vi "MGI Restore Front Panel Data.vi"(6 "Section Name (\"Data Values\")":string="Data Values", 7 "VI (Caller)":refnum<vi>, 8 "error in (no error)":errorcluster, 11 "Path":path) -> (0 "Error Out":errorcluster)   [LabVIEW 2020]
doc: "Restores the control and indicator data from the specified MGI Read/Write Anything file.\nControl and Indicator names must be unique.\n\nAuthored by Shawn Walpole\nsupport@mooregoodideas.com\nwww.mooregoodideas.com\n\nCopyright (c) 2010, Moore Good Ideas, Inc.\n\nAll rights reserved.\n\nRedistribution and use in source and binary forms, with or without modification, are permitted provided that the following conditions are met:\n\n * Redistributions of source code must retain the above copyright notice, this list of conditions and the following disclaimer.\n * Redistributions in binary form must reproduce the above copyright notice, this list of conditions and the following disclaimer in the documentation and/or other materials provided with the distribution.\n * Neither the name of Moore Good Ideas, Inc. nor the names of its contributors may be used to endorse or promote products derived from this software without specific prior written permission.\n\nTHIS SOFTWARE IS PROVIDED BY THE COPYRIGHT HOLDERS AND CONTRIBUTORS \"AS IS\" AND ANY EXPRESS OR IMPLIED WARRANTIES, INCLUDING, BUT NOT LIMITED TO, THE IMPLIED WARRANTIES OF MERCHANTABILITY AND FITNESS FOR A PARTICULAR PURPOSE ARE DISCLAIMED. IN NO EVENT SHALL THE COPYRIGHT OWNER OR CONTRIBUTORS BE LIABLE FOR ANY DIRECT, INDIRECT, INCIDENTAL, SPECIAL, EXEMPLARY, OR CONSEQUENTIAL DAMAGES (INCLUDING, BUT NOT LIMITED TO, PROCUREMENT OF SUBSTITUTE GOODS OR SERVICES; LOSS OF USE, DATA, OR PROFITS; OR BUSINESS INTERRUPTION) HOWEVER CAUSED AND ON ANY THEORY OF LIABILITY, WHETHER IN CONTRACT, STRICT LIABILITY, OR TORT (INCLUDING NEGLIGENCE OR OTHERWISE) ARISING IN ANY WAY OUT OF THE USE OF THIS SOFTWARE, EVEN IF ADVISED OF THE POSSIBILITY OF SUCH DAMAGE."
uses:
  <userlib>/_MGI/Application Control/MGI VI Reference/MGI Caller's VI Reference.vi
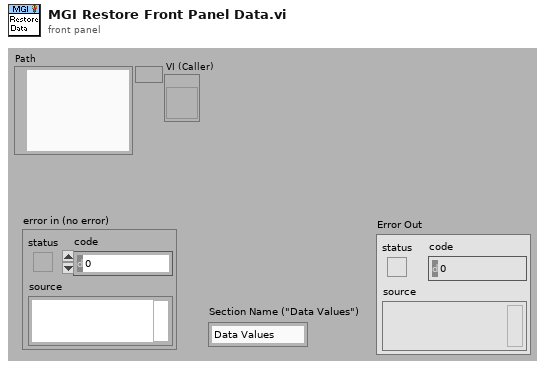
[diagram p1: front panel]
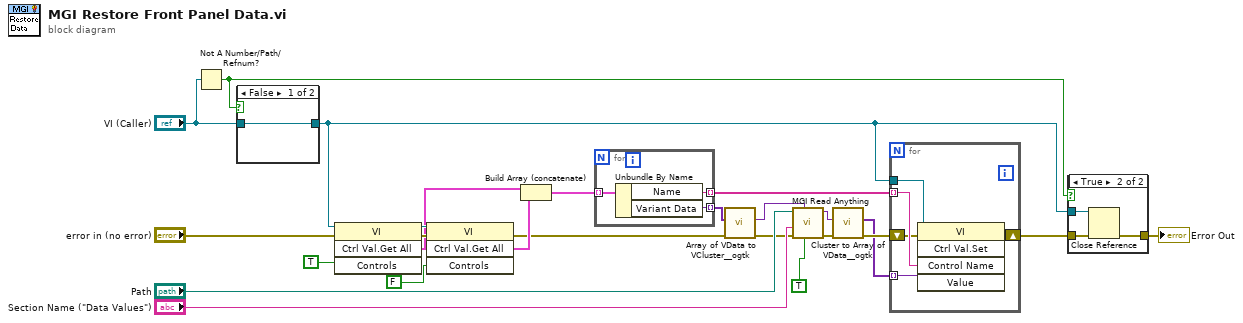
[diagram p0: block diagram]
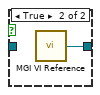
[diagram p3: hidden frame]
diagram:
  n1 = Not A Number/Path/Refnum?(number/path/refnum="VI (Caller)") -> (NaN/Path/Refnum?=w22:bool)
  n2 = case shown="False" w22 {
    tunnel: [w26 w27] -> w1
    tunnel: "VI (Caller)" -> [w26 _]
    frame False {
    }
    frame True {
      n3 = call-poly <userlib>:"MGI VI Reference.vi"() -> ("Caller's VI Reference"=w27:refnum<vi>)  [unwired: 1 in]
    }
  }
  n4 = invoke class="VI" method="Ctrl Val.Get All"(reference=w1, error in="error in (no error)", "Controls"=TRUE) -> (reference out=w18:refnum<vi>, error out=w17:errorcluster, "Get All Control Values Variant"=w16:cluster{"Name":string, "Variant Data":variant}[])  [unwired: 1 in, 1 out]
  n5 = invoke class="VI" method="Ctrl Val.Get All"(reference=w18, error in=w17, "Controls"=FALSE) -> (error out=w12:errorcluster, "Get All Control Values Variant"=w15:cluster{"Name":string, "Variant Data":variant}[])  [unwired: 1 in, 2 out]
  n6 = Build Array (concatenate)(w16, w15) -> (w11:cluster{"Name":string, "Variant Data":variant}[])
  n7 = for {
    tunnel: w11 -> [w29] mode=indexing
    tunnel: [w30] -> w3 mode=indexing
    tunnel: [w28] -> w9 mode=indexing
    n8 = Unbundle By Name(w29) -> ("Name"=w28:string, "Variant Data"=w30:variant)
  }
  n9 = call <userlib>:"Array of VData to VCluster__ogtk.vi"("error in (no error)"=w12, "Array"=w3) -> ("error out"=w4:errorcluster, "VCluster"=w5:variant)  [unwired: 8 in]
  n10 = call <userlib>:"MGI Read Anything.vi"("Use Supplied (F: Use Default)"=TRUE, "Type of Anything"=w5, "Error In"=w4, "Section Name (Name of \"Type of Anything\")"="Section Name (\"Data Values\")", "Path (dialog)"="Path") -> ("Error Out"=w6:errorcluster, "Anything"=w7:variant)  [unwired: 3 in, 2 out]
  n11 = call <userlib>:"Cluster to Array of VData__ogtk.vi"("error in (no error)"=w6, "Cluster"=w7) -> ("error out"=w10:errorcluster, "Array of VData"=w8:variant[])  [unwired: 8 in]
  n12 = for {
    tunnel: w8 -> [w34] mode=indexing
    tunnel: w9 -> [w35] mode=indexing
    shift-right: [w33] -> w21
    shift-left: w10 -> [w32]
    tunnel: w1 -> [w31]
    n13 = invoke class="VI" method="Ctrl Val.Set"(reference=w31, error in=w32, "Control Name"=w35, "Value"=w34) -> (error out=w33:errorcluster)  [unwired: 1 in, 4 out]
  }
  n14 = case shown="True" w22 {
    tunnel: w1 -> [_ w39]
    tunnel: w21 -> [w36 w38]
    tunnel: [w36 w37] -> w20
    frame False {
    }
    frame True {
      n15 = Close Reference(reference=w39, error in (no error)=w38) -> (error out=w37:errorcluster)
    }
  }
  "Error Out" <- w20
